vi "Identify.vi"(8 "error in (no error)":errorcluster, 11 "Laser Diode Controller in":refnum<class "KLD101.lvclass">) -> (0 "error out":errorcluster, 3 "Laser Diode Controller out":refnum<class "KLD101.lvclass">)   [LabVIEW 2016, in "Laser Diode Controller.lvlib" / "KLD101.lvclass"]
uses:
  KLD101.lvclass
  KLD101.lvclass/KLD101.ctl
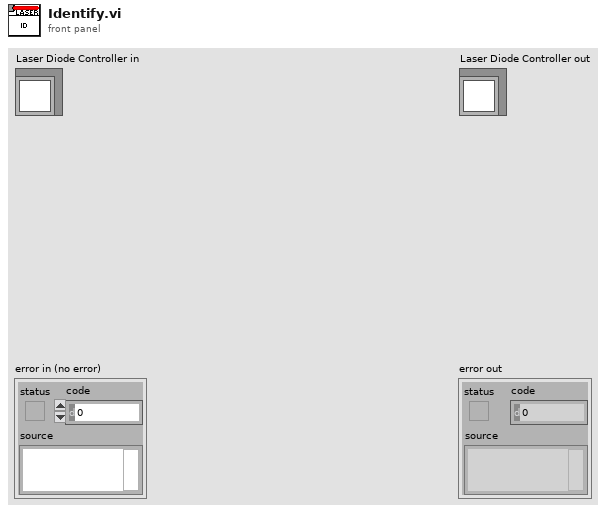
[diagram p1: front panel]
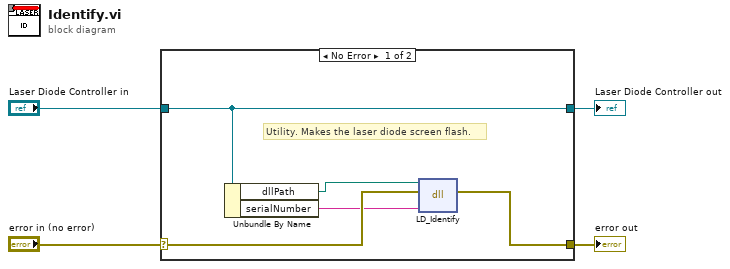
[diagram p0: block diagram]
diagram:
  n1 = case shown="No Error" "error in (no error)" {
    selector: "error in (no error)" -> [w8 w11]
    tunnel: [w7 w11] -> w3
    tunnel: [w9 w10] -> w1
    tunnel: "Laser Diode Controller in" -> [w9 w10]
    frame No Error {
      # "Utility. Makes the laser diode screen flash."
      n2 = Unbundle By Name(w9) -> ("dllPath"=w5:path, "serialNumber"=w6:string)
      n3 = dll-call lib="C:/IDEXX Software/Collimation/data/Thorlabs.MotionControl.KCube.LaserDiode.dll" fn="LD_Identify"(path in=w5, error in=w8, "serialNumber"=w6) -> (error out=w7:errorcluster)  [unwired: 3 in, 1 out]
    }
    frame Error {
    }
  }
  "error out" <- w3
  "Laser Diode Controller out" <- w1
